vi "Evaluate Value Change Trigger (Array).vi"(8 "error in (no error)":errorcluster, 10 "Trigger Data":dbl[](array[numeric]), 11 "Value Change Trigger in":refnum<class "Value Change Trigger.lvclass">) -> (0 "error out":errorcluster, 1 "Trigger indices":i32[](array[numeric]), 2 "Trigger":bool, 3 "Value Change Trigger out":refnum<class "Value Change Trigger.lvclass">)   [LabVIEW 2015, in "Value Change Trigger.lvclass"]
uses:
  Value Change Trigger.lvclass
  Value Change Trigger.lvclass/Value Change Trigger.ctl
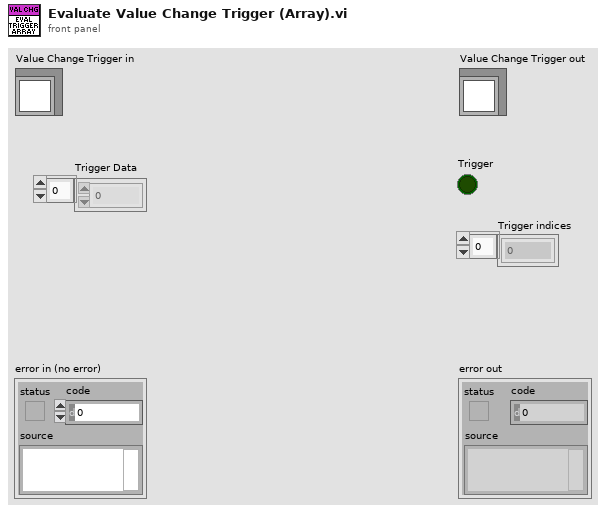
[diagram p1: front panel]
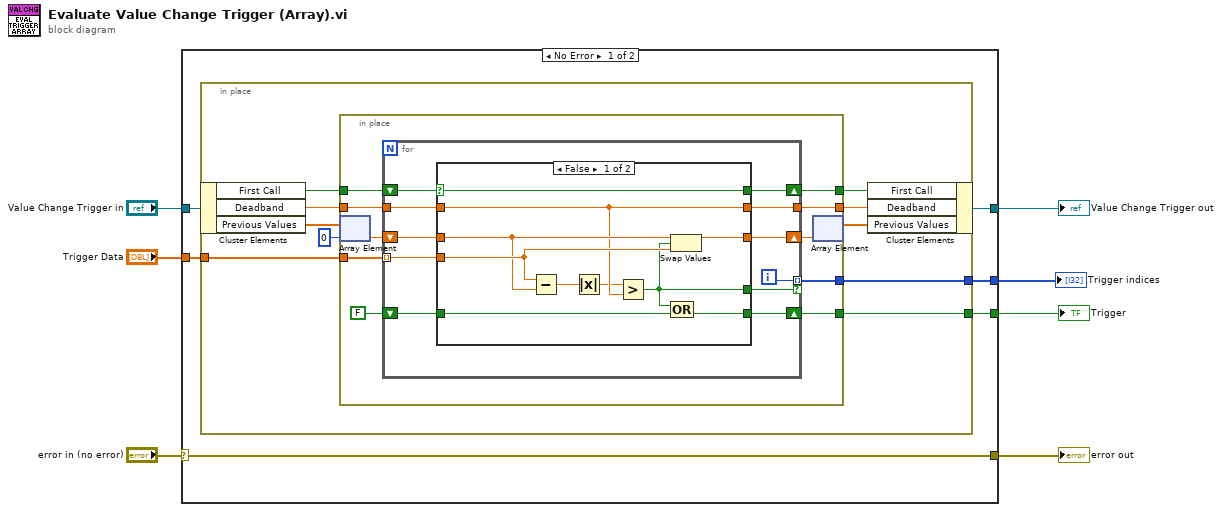
[diagram p0: block diagram]
diagram:
  n1 = case shown="No Error" "error in (no error)" {
    selector: "error in (no error)" -> [w9 w58]
    tunnel: "Value Change Trigger in" -> [w13 w59]
    tunnel: [w12 w59] -> w6
    tunnel: "Trigger Data" -> [w11 _]
    tunnel: [w10 _] -> w4
    tunnel: [w9 w58] -> w2
    tunnel: [w8 _] -> w1
    frame No Error {
      n2 = in-place {
        in-place-border: w11 -> [w19]
        in-place-border: [w22] -> w10
        in-place-border: [w14] -> w8
        n3 = in-place-cluster #1(w13) -> ("First Call"=w23:bool, "Deadband"=w20:dbl, "Previous Values"=w17:dbl[])
        n4 = in-place {
          in-place-border: w23 -> [w33]
          in-place-border: [w25] -> w22
          in-place-border: [w32] -> w21
          in-place-border: w20 -> [w31]
          in-place-border: w19 -> [w30]
          in-place-border: [w29] -> w18
          in-place-border: [w24] -> w14
          n5 = in-place-array #2(w17, 0) -> (w28:dbl)
          n6 = for {
            tunnel: [w42] -> w32
            tunnel: w31 -> [w41]
            tunnel: w30 -> [w40] mode=indexing
            shift-right: [w39] -> w29
            shift-left: w33 -> [w44]
            shift-right: [w38] -> w27
            shift-left: w28 -> [w43]
            shift-right: [w36] -> w25
            shift-left: FALSE -> [w37]
            tunnel: [w35] -> w24 mode=indexing if=w34
            i -> [w35]
            n7 = case shown="False" w44 {
              selector: w44 -> [w49 _]
              tunnel: w43 -> [w52 _]
              tunnel: [w53 w56] -> w38
              tunnel: w40 -> [w54 w56]
              tunnel: [w51 w55] -> w36
              tunnel: [w50 w57] -> w42
              tunnel: w41 -> [w50 w57]
              tunnel: [w49 _] -> w39
              tunnel: w37 -> [w48 w55]
              tunnel: [w45 _] -> w34
              frame False {
                n8 = Subtract(x=w54, y=w52) -> (x-y=w46:dbl)
                n9 = Absolute Value(x=w46) -> (abs(x)=w47:dbl)
                n10 = Greater?(x=w47, y=w50) -> (0:w45:bool)
                n11 = Swap Values(12:w52, 13:w45, 14:w54) -> (1:w53:dbl)  [unwired: 1 out]
                n12 = Compound Arithmetic op=OR(w45, w48) -> (w51:bool)
              }
              frame True {
                # "Just latch the trigger channel values on first call."
              }
            }
          }
          n13 = in-place-array #2(w27) -> (w15:dbl[])  [unwired: 1 out]
        }
        n14 = in-place-cluster #1("First Call"=w18, "Deadband"=w21, "Previous Values"=w15) -> (w12:refnum<class "Value Change Trigger.lvclass">)
      }
    }
    frame Error {
    }
  }
  "error out" <- w2
  "Value Change Trigger out" <- w6
  "Trigger" <- w4
  "Trigger indices" <- w1
